vi "VescTestV2.vi"() -> ()   [LabVIEW 2019]
uses:
  <vilib>/myRIO/Instrument Drivers/Onboard IO/UART/typedef/VISA Configuration.ctl
  <vilib>/Instr/_visa.llb/VISA Configure Serial Port (Instr).vi
  <vilib>/myRIO/Express VI/Onboard IO/UART/UART Express VI.xnode
  <vilib>/myRIO/Instrument Drivers/Onboard IO/UART/UART.lvlib
  usr/local/lib/libvescEncoder.so
panel:
  in  "stop":bool
  in  "Current":u16
  out "Numeric":dbl
  out "TX":string
  out "Command":dbl[](array[numeric])
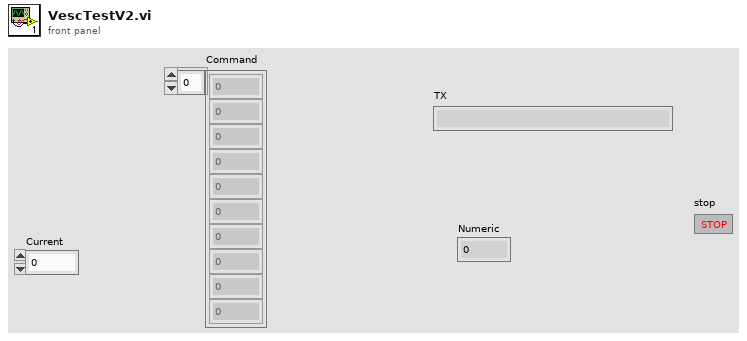
[diagram p1: front panel]
types:
  T1 = typedef "UART.lvlib/VISA Configuration.ctl" = cluster{"baud rate (9600)":u32, "data bits (8)":u16, "parity (0:none)":enum16{"None", "Odd", "Even", "Mark", "Space"}, "stop bits (10: 1 bit)":u16, "flow control (0:none)":u16, "termination char\n(0xA = '\\n' = LF) ":u8, "Enable Termination\nChar (T)":bool, "timeout (10sec)":u32}
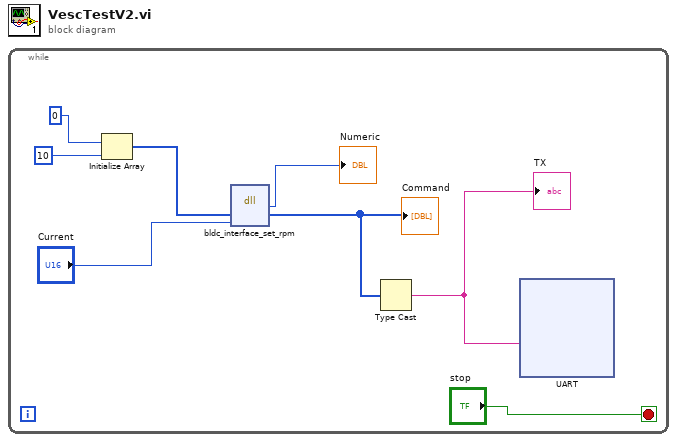
[diagram p0: block diagram]
diagram:
  n1 = while {
    stop <- "stop" stop-if-true
    n2 = Initialize Array(0, 10) -> (w7:i32[])
    n3 = dll-call lib="usr/local/lib/libvescEncoder.so" fn="bldc_interface_set_rpm"("array"=w7, "rpm"="Current") -> ("return type"=→"Numeric":i32, "array"=w8:u8[])  [unwired: 4 in, 2 out]
    "Command" <- w8
    n4 = Type Cast(x=w8) -> (*(type *) &x=w3:string)  [unwired: 1 in]
    "TX" <- w3
    n5 = xnode "UART"("Characters to Write"=w3) -> ()  [unwired: 1 in, 2 out]
  }
